vi "Mecanum PID.vi"() -> ()   [LabVIEW 2014]
uses:
  <vilib>/Rock Robotics/WPI/CAN/TalonSRX/WPI_CANTalonSRX_APIControlMode.ctl
  <vilib>/Rock Robotics/WPI/CAN/TalonSRX/WPI_CANTalonSRX_APIFeedbackSelect.ctl
  <vilib>/Rock Robotics/WPI/MotorControl/WPI_MotorControlOpenCANTalonSRX.vi
panel:
  in  "I":dbl
  in  "F":dbl=0.01
  in  "D":dbl
  in  "P":dbl=1.0
  in  "Reverse Feedback Sensor":bool
  in  "Slave Device Number":u8=1
  in  "Encoder Codes Per Rev":u16=360
  in  "Master Device Number":u8
  in  "stop":bool
  in  "Set Speed (RPM)":dbl(slide) scale=-2500.0..2500.0
  out "Actual Speed (RPM)":dbl(knob) scale=-2500.0..2500.0 scale format="%4d"
  out "Feedback Chart":cluster{dbl, dbl}(graph)
  # "roboRIO Wiring Diagram"
  # "Slave Talon SRX"
  # "Master Talon SRX"
  # "Gnd"
  # "A"
  # "B"
  # "+5V"
  # "US Digital E4P Encoder"
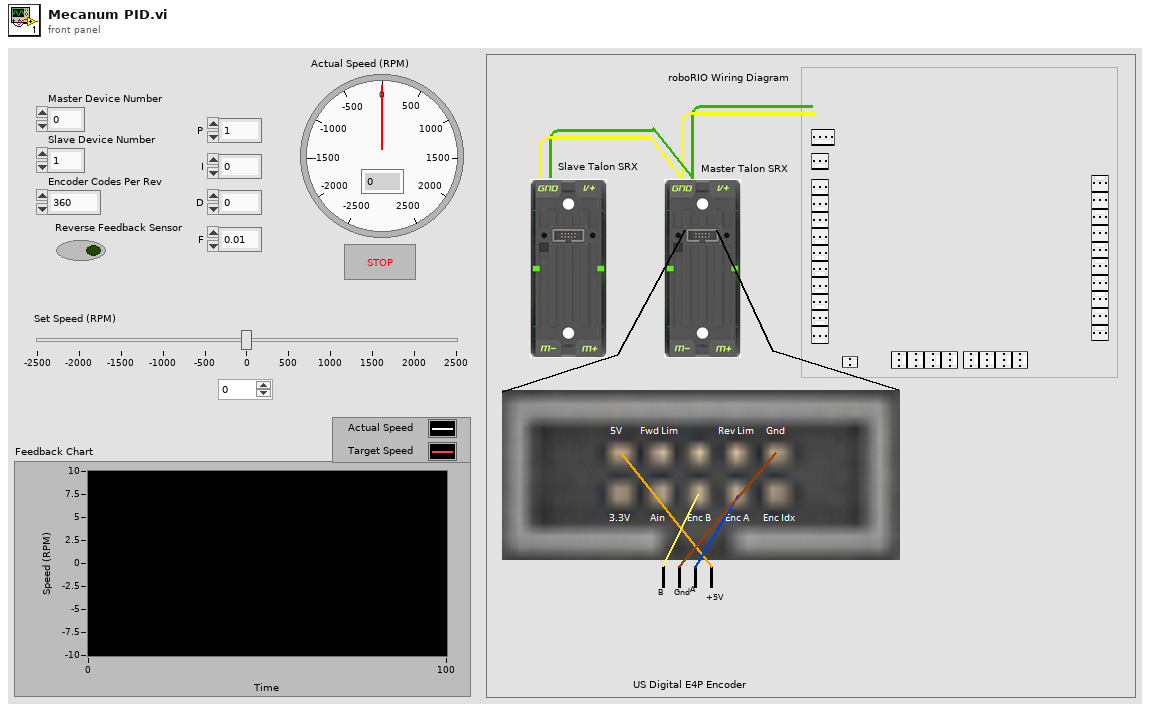
[diagram p1: front panel]
types:
  T1 = typedef "WPI_CANTalonSRX_APIControlMode.ctl" = enum8{"Percent VBus", "Speed", "Position", "Slave", "Unchanged / Invalid"}
  T2 = typedef "WPI_CANTalonSRX_APIFeedbackSelect.ctl" = enum16{"Digital Quadrature Encoder", "Analog Potentiometer", "Analog Encoder"}
  T3 = typedef "WPI_MotorControlDeviceRef.ctl" = cluster{"DeviceStatus":errorcluster, "Type":T4, "PWM":cluster{"Controller":T5, "PWM Channel":T6, "DeadBand":T7}, "CAN":cluster{"Device Number":u8, "Control Mode":T8, "Semaphore":T9, "Max Vout":dbl, "TalonSRX Control Mode":T1}, "Invert":bool, "TransformRef":T10, "InvTransformRef":T10}
  T4 = typedef "WPI_MotorControlType.ctl" = enum16{"PWM", "CAN", "CANTalonSRX"}
  T5 = typedef "FPGA_TypedefDigitalModule.ctl" = enum16{"Controller 1"}
  T6 = typedef "FPGA_DIOPWMChannel.ctl" = enum8{"PWM 0", "PWM 1", "PWM 2", "PWM 3", "PWM 4", "PWM 5", "PWM 6", "PWM 7", "PWM 8", "PWM 9", "PWM MXP 0", "PWM MXP 1", "PWM MXP 2", "PWM MXP 3", "PWM MXP 4", "PWM MXP 5", "PWM MXP 6", "PWM MXP 7", "PWM MXP 8", "PWM MXP 9", "Invalid"}
  T7 = typedef "WPI_PWMDeadband.ctl" = cluster{"Name":string, "maxPositivePwm":i32, "minPositivePwm":i32, "centerPwm":i32, "maxNegativePwm":i32, "minNegativePwm":i32, "angularRange":u16}
  T8 = typedef "WPI_CANJaguar_ControlMode.ctl" = enum8{"Percent VBus", "Current", "Speed", "Position", "Voltage"}
  T9 = typedef "Semaphore RefNum" = refnum<k1>
  T10 = typedef "WPI_PWMTransform_ConPane.ctl" = refnum<vi>
  T11 = typedef "WPI_CANTalonSRX_GlobalStatus.ctl" = cluster{"Applied Throttle":dbl, "Module Enabled":bool, "CAN Error":errorcluster, "Closed Loop Error":dbl, "Forward Limit Switch Closed":bool, "Reverse Limit Switch Closed":bool, "Sensor Position":dbl, "Sensor Velocity":dbl, "Current":dbl, "Sticky Fault - Over Temp":bool, "Sticky Fault - Under Voltage":bool, "Sticky Fault - Forward Limit":bool, "Sticky Fault - Reverse Limit":bool, "Sticky Fault - Forward Soft Limit":bool, "Sticky Fault - Reverse Soft Limit":bool, "Brake is Enabled":bool, "Encoder Position":dbl, "Encoder Velocity":dbl, "Encoder Index Count":dbl, "Encoder A Pin State":bool, "Encoder B Pin State":bool, "Encoder Index Pin State":bool, "Analog In":dbl, "Analog In Velocity":dbl, "Temperature (C)":dbl, "Battery Voltage":dbl}
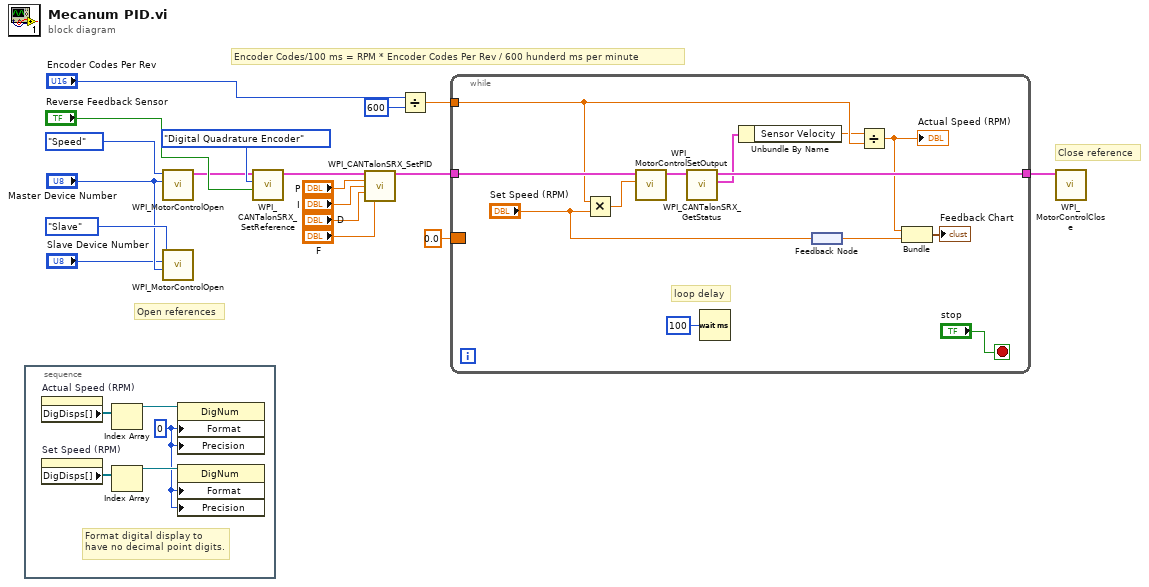
[diagram p0: block diagram]
diagram:
  # "Encoder Codes/100 ms = RPM * Encoder Codes Per Rev / 600 hunderd ms per minute"
  # "Open references"
  # "Close reference"
  n1 = stacked-sequence {
    frame #0 {
      w19 = u8 0 ("Display Format:Format")
      # "Format digital display to have no decimal point digits."
      n2 = property on="Actual Speed (RPM)" class="Knob (strict)"() -> ("DigDisps[]"=w23:refnum<vi>[])  [unwired: 2 in, 2 out]
      n3 = property on="Set Speed (RPM)" class="Slide (strict)"() -> ("DigDisps[]"=w20:refnum<vi>[])  [unwired: 2 in, 2 out]
      n4 = Index Array(array=w23) -> (element=w22:refnum<vi>)  [unwired: 1 in]
      n5 = Index Array(array=w20) -> (element=w21:refnum<vi>)  [unwired: 1 in]
      n6 = property class="DigNum"(reference=w22, "Format"=w19, "Precision"=w19) -> ()  [unwired: 1 in, 2 out]
      n7 = property class="DigNum"(reference=w21, "Format"=w19, "Precision"=w19) -> ()  [unwired: 1 in, 2 out]
    }
  }
  n8 = call-poly <vilib>:"WPI_MotorControlOpen.vi"("Device Number"="Master Device Number", "Control Mode"=WPI_CANTalonSRX_APIControlMode."Speed") -> ("MotorControlDeviceRef"=w4:T3)  [unwired: 5 in, 4 out]
  n9 = call-poly <vilib>:"WPI_MotorControlOpen.vi"("Master Device Number"="Master Device Number", "Device Number"="Slave Device Number", "Control Mode"=WPI_CANTalonSRX_APIControlMode."Slave") -> ()  [unwired: 4 in, 5 out]
  n10 = call <vilib>:"WPI_CANTalonSRX_SetReference.vi"("Reverse Feedback Sensor"="Reverse Feedback Sensor", "Feedback Reference"=WPI_CANTalonSRX_APIFeedbackSelect."Digital Quadrature Encoder", "CAN Talon SRX Ref"=w4) -> ("CAN Talon SRX Ref Out"=w3:T3)  [unwired: 7 in, 1 out]
  n11 = call <vilib>:"WPI_CANTalonSRX_SetPID.vi"("CAN Talon SRX Ref"=w3, "P"="P", "I"="I", "D"="D", "F"="F") -> ("CAN Talon SRX Ref Out"=w17:T3)  [unwired: 9 in, 1 out]
  n12 = Divide(x="Encoder Codes Per Rev", y=u16 600) -> (x/y=w13:dbl)
  n13 = while {
    tunnel: w17 -> [w34]
    tunnel: [w33] -> w18
    tunnel: w13 -> [w32]
    border: 0.0 -> [_]
    stop <- "stop" stop-if-true
    # "loop delay"
    n14 = Multiply(x=w32, y="Set Speed (RPM)") -> (x*y=w28:dbl)
    n15 = call <vilib>:"WPI_MotorControlSetOutput.vi"("Output"=w28, "MotorControlDevRef"=w34) -> ("MotorControlDevRef"=w31:T3)  [unwired: 7 in, 2 out]
    n16 = call <vilib>:"WPI_CANTalonSRX_GetStatus.vi"("CAN Talon SRX Ref"=w31) -> ("Talon SRX Status"=w30:T11, "CAN Talon SRX Ref Out"=w33:T3)  [unwired: 8 in, 1 out]
    n17 = Wait (ms)(milliseconds to wait=u32 100) -> ()  [unwired: 1 out]
    n18 = Unbundle By Name(w30) -> ("Sensor Velocity"=w29:dbl)
    n19 = feedback #1() -> (w26:dbl)
    n20 = feedback-in #1("Set Speed (RPM)") -> ()
    n21 = Divide(x=w29, y=w32) -> (x/y=w27:dbl)
    "Actual Speed (RPM)" <- w27
    n22 = Bundle(w27, w26) -> (→"Feedback Chart":cluster{dbl, dbl})  [unwired: 1 in]
  }
  n23 = call <vilib>:"WPI_MotorControlClose.vi"("MotorControlDevRef"=w18) -> ()  [unwired: 10 in, 1 out]
